vi "ConvertStrTimeToTimeStamp.vi"(10 "type":enum16{"년(2)-월(2)-일(2) 시-분-초"}(ring), 11 "date/time string":string) -> (3 "TimeStamp":timestamp)   [LabVIEW 2018, in "Library-DataConvert.lvlib"]
uses:
  Library-DataConvert.lvlib
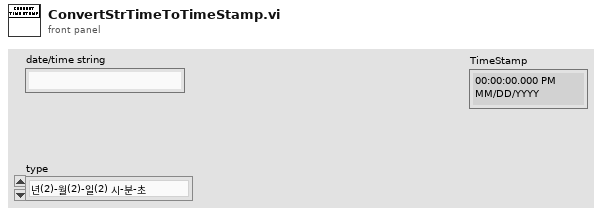
[diagram p1: front panel]
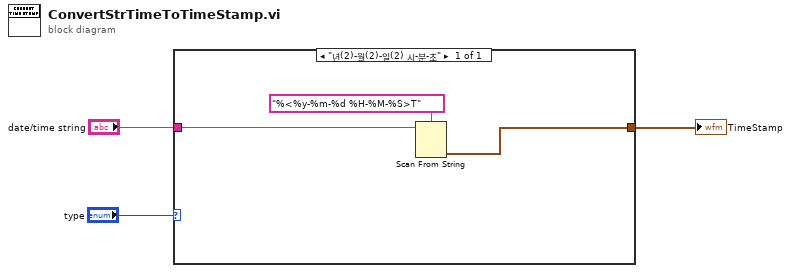
[diagram p0: block diagram]
diagram:
  n1 = case shown="\"년(2)-월(2)-일(2) 시-분-초\"" "type" {
    tunnel: "date/time string" -> [w5]
    tunnel: [w4] -> w1
    frame "년(2)-월(2)-일(2) 시-분-초" {
      n2 = Scan From String(format string="%<%y-%m-%d %H-%M-%S>T" ("포맷 문자열"), input string=w5) -> (output 1=w4:timestamp)  [unwired: 3 in, 3 out]
    }
  }
  "TimeStamp" <- w1
